vi "Pfeiffer Vacuum MiniTest Measure.vi"(8 "error in (no error)":errorcluster, 9 "MiniTest Measure - Cluster":T1={"Parameter"=3, "Parameter\nread only<->describe"=FALSE, "Value in"=1e-09} {"Value in" min=1e-09 max=100000.0 step=1e-09 format="%.2e"; "Parameter" items=[" Pressure of the ext. Gauge [mbar] (read only)", " Zero (update background suppression)", " Leakrate [selected unit] (read only)", " Leakrate  [mbarl/s] (read only)", " Leakrate of external test leak [selected unit] (read only)", " Pressure internal sensor [selected unit] (read only)", " Trigger [selected unit]", " Trigger [mbar l/s]", " Pressure of the ext. Gauge [selected unit] (read only]", " Gauge Type (read only)"]}, 10 "Adress of unit":u16=1 min=1 max=999 step=1, 11 "COM Port Name in":refnum<visa-resource-name>="COM1") -> (0 "error out":errorcluster, 2 "response (data)":string)   [LabVIEW 2021]
doc: "This VI is an example of how to use the Pfeiffer Vacuum subVIs programmatically. This VI first initializes the instrument, takes measurements, then closes the instrument."
uses:
  <instrlib>/Pfeiffer Vacuum/Public/MiniTest/PV MiniTest Measure - Cluster.ctl
  <instrlib>/Pfeiffer Vacuum/Pfeiffer Vacuum.lvlib
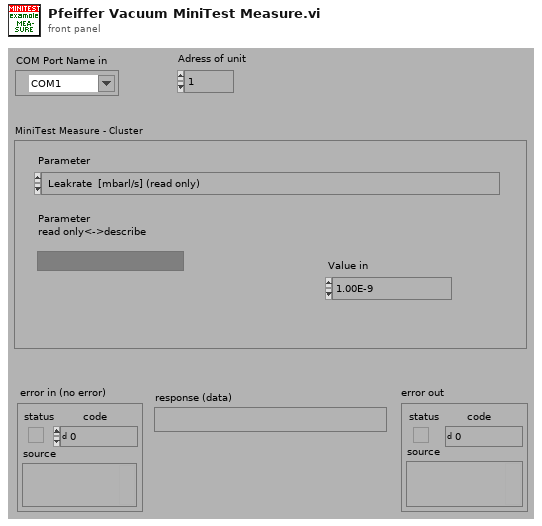
[diagram p1: front panel]
types:
  T1 = typedef "Pfeiffer Vacuum.lvlib/PV MiniTest Measure - Cluster.ctl" = cluster{"Parameter":u16, "Parameter\nread only<->describe":bool, "Value in":dbl}
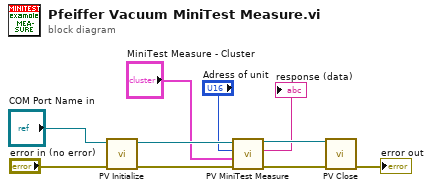
[diagram p0: block diagram]
diagram:
  n1 = call <instrlib>:"PV Initialize.vi"("error in (no error)"="error in (no error)", "VISA session in"="COM Port Name in") -> ("error out"=w10:errorcluster, "VISA session out"=w8:refnum<visa-resource-name>)  [unwired: 8 in]
  n2 = call <instrlib>:"PV MiniTest Measure.vi"("error in (no error)"=w10, "MiniTest Measure - Cluster"="MiniTest Measure - Cluster", "Adress of unit"="Adress of unit", "VISA session"=w8) -> ("error out"=w9:errorcluster, "response (data)"=→"response (data)":string, "dup VISA session"=w7:refnum<visa-resource-name>)  [unwired: 5 in]
  n3 = call <instrlib>:"PV Close.vi"("VISA session"=w7, "error in (no error)"=w9) -> ("error out"=→"error out":errorcluster)  [unwired: 13 in]
